vi "Draw Depth Frame.vi"(8 "Error In":errorcluster, 10 "U16 Array":u8[](array[numeric]), 11 "Image":T1) -> (0 "Error Out":errorcluster, 3 "Image Out":T1)   [LabVIEW 2011, in "LVH-KinectOne.lvlib"]
doc: "Converts the Depth data to a Greyscale U16 IMAQ Image."
uses:
  LVH-KinectOne.lvlib
  <vilib>/vision/Image Controls.llb/IMAQ Image.ctl
  Private/Frame Description FGV [Depth].vi
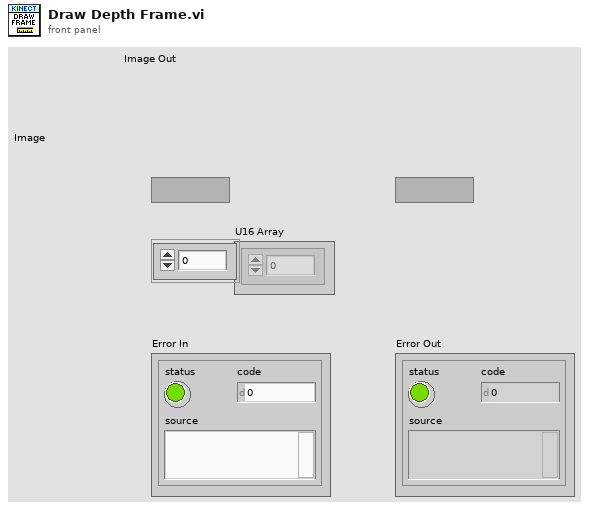
[diagram p1: front panel]
types:
  T1 = typedef "IMAQ Image.ctl" = refnum<image>
  T2 = typedef "LVH-KinectOne.lvlib/FrameDescription.ctl" = cluster{"BytesPerPixel":u32, "DiagonalFieldOfView":sgl, "Height":i32, "HorizontalFieldOfView":sgl, "LengthInPixels":u32, "VerticalFieldOfView":sgl, "Width":i32}
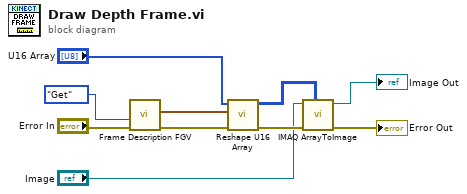
[diagram p0: block diagram]
diagram:
  n1 = call-poly "Frame Description FGV.vi"("error in (no error)"="Error In", "Command"=enum16{"Get", "Set"}."Get") -> ("error out"=w10:errorcluster, "FrameDescription"=w8:T2)  [unwired: 8 in]
  n2 = call "Reshape U16 Array.vi"("error in (no error)"=w10, "FrameDescription"=w8, "U16 Array"="U16 Array") -> ("error out"=w7:errorcluster, "2D Array"=w6:u16[][])  [unwired: 7 in]
  n3 = call "IMAQ ArrayToImage"("Image Pixels (U16)"=w6, "error in (no error)"=w7, "Image"="Image") -> ("error out"=→"Error Out":errorcluster, "Image Out"=→"Image Out":T1)  [unwired: 7 in]
